vi "HH_FIFORead.vi"(0 "Device Index":i32, 5 "Buffer In":u32[](array[numeric]), 7 "Count":i32, 11 "error in (no error)":errorcluster) -> (4 "OK":bool, 6 "Buffer Out":u32[](array[numeric]), 8 "Data Count":i32, 14 "FiFo Overrun":bool, 15 "error out":errorcluster)   [LabVIEW 2009]
uses:
  newCore/MT Scan/SubVIs/hhlib.dll
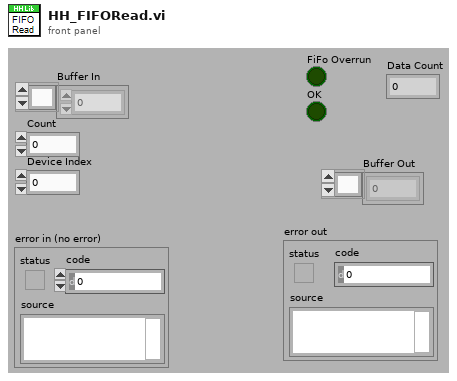
[diagram p1: front panel]
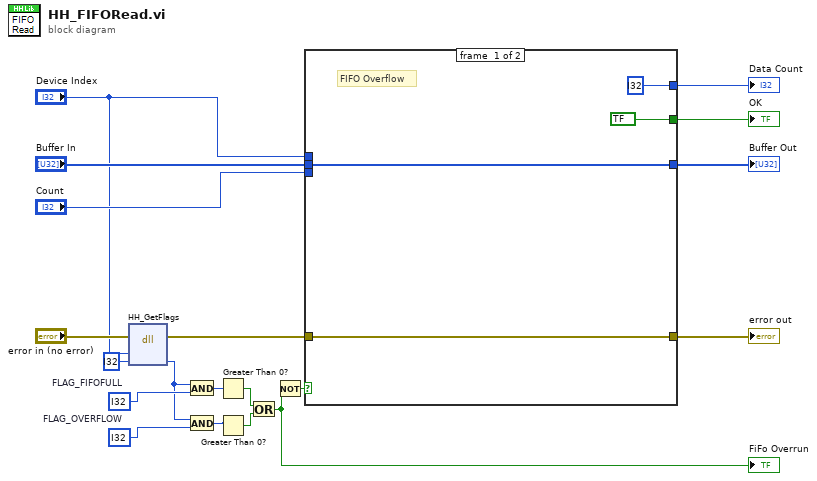
[diagram p0: block diagram]
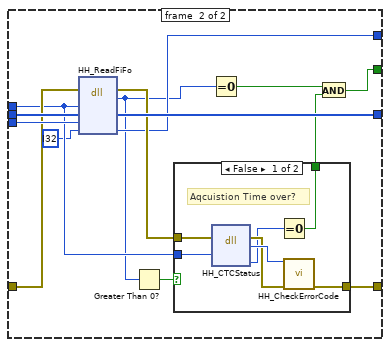
[diagram p2: hidden frame]
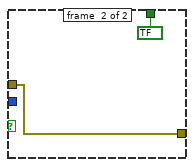
[diagram p3: hidden frame]
diagram:
  w5 = i32 ?  # FLAG_OVERFLOW
  w15 = i32 ?  # FLAG_FIFOFULL
  n1 = dll-call lib="C:/Users/dhaehnel/Documents/Workspace/Labview_Workspace/newCore/MT Scan/SubVIs/hhlib.dll" fn="HH_GetFlags"(error in="error in (no error)", "devidx"="Device Index", "flags"=i32 ?) -> (error out=w12:errorcluster, "flags"=w6:i32)  [unwired: 4 in, 1 out]
  n2 = And(x=w6, y=w15) -> (x .and. y?=w14:i32)
  n3 = And(x=w6, y=w5) -> (x .and. y?=w7:i32)
  n4 = Greater Than 0?(x=w14) -> (x > 0?=w4:bool)
  n5 = Greater Than 0?(x=w7) -> (x > 0?=w3:bool)
  n6 = Or(x=w4, y=w3) -> (x .or. y?=w2:bool)
  "FiFo Overrun" <- w2
  n7 = Not(x=w2) -> (.not. x?=w1:bool)
  n8 = case shown="True" w1 {
    tunnel: "Buffer In" -> [w21 w37]
    tunnel: "Count" -> [_ w36]
    tunnel: "Device Index" -> [_ w30]
    tunnel: [bool ? ("OK") w32] -> w13
    tunnel: w12 -> [w22 w35]
    tunnel: [w22 w27] -> w11
    tunnel: [w21 w34] -> w10
    tunnel: [i32 ? ("return type") w25] -> w9
    frame #0 {
      # "FIFO Overflow"
    }
    frame #1 {
      n9 = dll-call lib="C:/Users/dhaehnel/Documents/Workspace/Labview_Workspace/newCore/MT Scan/SubVIs/hhlib.dll" fn="HH_ReadFiFo" label="PH_TTReadData"(error in=w35, "devidx"=w30, "buffer"=w37, "count"=w36, "nactual"=i32 ?) -> (error out=w29:errorcluster, "return type"=w24:i32, "buffer"=w34:u32[], "nactual"=w25:i32)  [unwired: 4 in, 1 out]
      n10 = Greater Than 0?(x=w24) -> (x > 0?=w31:bool)
      n11 = case shown="False" w31 {
        tunnel: w30 -> [w44 _]
        tunnel: w29 -> [w43 w45]
        tunnel: [w42 bool ?] -> w28
        tunnel: [w39 w45] -> w27
        frame #0 {
          # "Aqcuistion Time over?"
          n12 = dll-call lib="C:/Users/dhaehnel/Documents/Workspace/Labview_Workspace/newCore/MT Scan/SubVIs/hhlib.dll" fn="HH_CTCStatus" label="PH_CTCStatus"(error in=w43, "devidx"=w44) -> (error out=w40:errorcluster, "return type"=w41:i32, "ctcstatus"=w38:i32)  [unwired: 4 in, 1 out]
          n13 = Equal To 0?(x=w38) -> (x = 0?=w42:bool)
          n14 = call "HH_CheckErrorCode.vi"("errcode"=w41, "error in (no error)"=w40) -> ("error out"=w39:errorcluster)  [unwired: 12 in, 1 out]
        }
        frame #1 {
        }
      }
      n15 = Equal To 0?(x=w24) -> (x = 0?=w33:bool)
      n16 = And(x=w33, y=w28) -> (x .and. y?=w32:bool)
    }
  }
  "OK" <- w13
  "error out" <- w11
  "Buffer Out" <- w10
  "Data Count" <- w9
